vi "WSVCAP SHL Host TL SPI_RFFE Query Cycle Count.vi"(11 "error in":errorcluster) -> (4 "Cycle Count":u64, 15 "error out":errorcluster)   [LabVIEW 2012]
uses:
  Type Defs/WSVCAP SHL Top Level Control Operation Enum.ctl
  Type Defs/WSVCAP SHL Top Level Control Enum.ctl
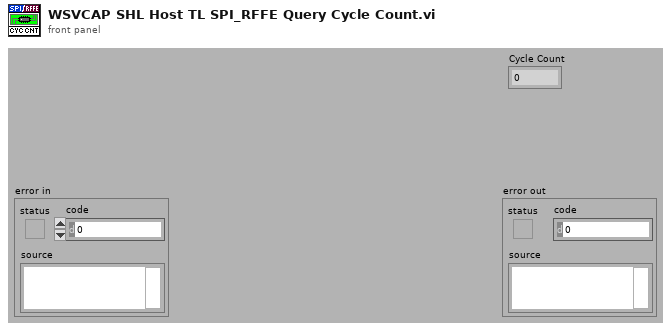
[diagram p1: front panel]
types:
  T1 = typedef "WSVCAP SHL Top Level Control Enum.ctl" = enum16{"Start", "Cmd", "Transaction", "Wait Ticks", "Socket Mask", "Slave Address", "Sub Address", "Bytes to Write", "Bytes to Read", "Write Data", "Write Flag", "Read Data", "Read Flag", "Ack Read", "Read Status Flag", "Ack Read Status", "Status", "Cycle Count", "Stop Cycle", "Exit"}
  T2 = typedef "WSVCAP SHL Top Level Control Operation Enum.ctl" = enum16{"Initialize", "Set Control", "Read Control", "Close"}
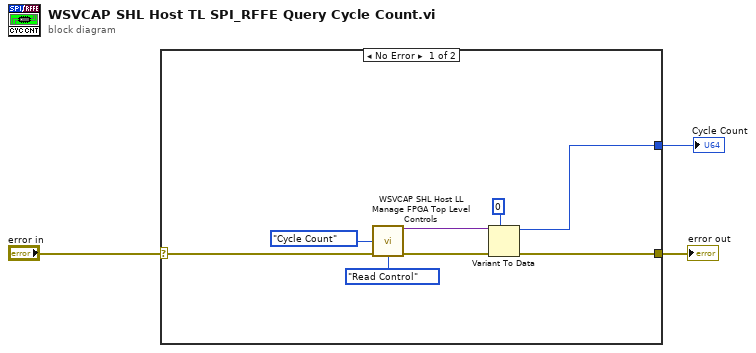
[diagram p0: block diagram]
diagram:
  n1 = case shown="No Error" "error in" {
    selector: "error in" -> [w9 _]
    tunnel: [w7 _] -> w3
    tunnel: [w4 _] -> w1
    frame No Error {
      n2 = call "WSVCAP SHL Host LL Manage FPGA Top Level Controls.vi"("FPGA Top Level Control"=WSVCAP_SHL_Top_Level_Control_Enum."Cycle Count", "error in (no error)"=w9, "Operation"=WSVCAP_SHL_Top_Level_Control_Operation_Enum."Read Control") -> ("Value Out"=w6:variant, "error out"=w8:errorcluster)  [unwired: 11 in]
      n3 = Variant To Data(error in=w8, type=u64 0, Variant=w6) -> (data=w4:u64, error out=w7:errorcluster)
    }
    frame Error {
    }
  }
  "error out" <- w3
  "Cycle Count" <- w1
